vi "EndTest_SameTest_ReturnsNoError.vi"() -> (0 "error out":errorcluster)   [LabVIEW 2017, in "ResultTreeListener.Tests.lvlib"]
uses:
  ResultTreeListener.Tests.lvlib
  Support/FakeTestCase/FakeTestCase.lvclass
  C:/Users/de200256/Code/logmanoriginal/lvunit/Test/Test.lvclass
  ResultTreeListener/ResultTreeListener.lvclass
  ResultTree/ResultTree.lvclass
  Assertion/Assertion.lvlib
panel:
  in  "Tree":string(tree)
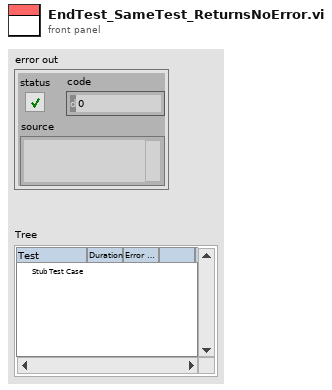
[diagram p1: front panel]
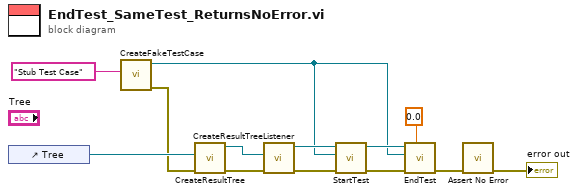
[diagram p0: block diagram]
diagram:
  n1 = control-ref of="Tree"() -> (w7:refnum<vi>)
  n2 = call "CreateFakeTestCase.vi"("Name"="Stub Test Case") -> ("error out"=w4:errorcluster, "FakeTestCase out"=w2:refnum<class "FakeTestCase.lvclass">)  [unwired: 9 in]
  n3 = call "CreateResultTree.vi"("error in (no error)"=w4, "Tree Refnum"=w7) -> ("error out"=w13:errorcluster, "ResultTree out"=w12:refnum<class "ResultTree.lvclass">)  [unwired: 8 in]
  n4 = call "CreateResultTreeListener.vi"("error in (no error)"=w13, "ResultTree"=w12) -> ("error out"=w11:errorcluster, "ResultTreeListener out"=w9:refnum<class "ResultTreeListener.lvclass">)  [unwired: 8 in]
  n5 = call-dynamic "StartTest.vi"("error in (no error)"=w11, "Test"=w2, "ResultTreeListener in"=w9) -> ("error out"=w6:errorcluster, "ResultTreeListener out"=w5:refnum<class "ResultTreeListener.lvclass">)  [unwired: 7 in]
  n6 = call-dynamic "EndTest.vi"("Time"=0.0, "error in (no error)"=w6, "Test"=w2, "ResultTreeListener in"=w5) -> ("error out"=w3:errorcluster)  [unwired: 6 in, 1 out]
  n7 = call "Assert No Error.vi"("error in (no error)"=w3) -> ("error out"=→"error out":errorcluster)  [unwired: 10 in]
